vi "Seconds to Time String.vi"(11 "Seconds":dbl format="%#_13g") -> (3 "Time String":string)   [LabVIEW 2013]
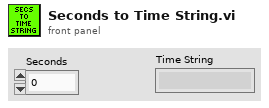
[diagram p1: front panel]
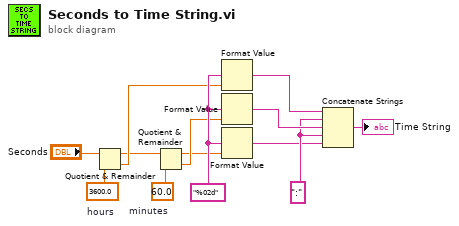
[diagram p0: block diagram]
diagram:
  w13 = "%02d" ("format string")
  w7 = ":"
  w4 = 3600.0  # hours
  w5 = 60.0  # minutes
  n1 = Quotient & Remainder(x="Seconds", y=w4) -> (x-y*floor(x/y)=w3:dbl, floor(x/y)=w11:dbl)
  n2 = Quotient & Remainder(x=w3, y=w5) -> (x-y*floor(x/y)=w10:dbl, floor(x/y)=w12:dbl)
  n3 = Format Value(format string=w13, value (0)=w11) -> (output string=w9:string)  [unwired: 1 in]
  n4 = Format Value(format string=w13, value (0)=w12) -> (output string=w8:string)  [unwired: 1 in]
  n5 = Format Value(format string=w13, value (0)=w10) -> (output string=w6:string)  [unwired: 1 in]
  n6 = Concatenate Strings(w9, w7, w8, w7, w6) -> (→"Time String":string)
